vi "PmuError.vi"(8 "error in (no error)":errorcluster, 10 "clPmuImpairRptArray":T1 {"Synx" format="%#_4g"}, 11 "clEvtReportArray":T1 {"Synx" format="%#_4g"}) -> (0 "error out":errorcluster, 3 "Results":dbl[][](array[numeric]))   [LabVIEW 2017, in "OutputToFilePlugins.lvlib" / "OutputToFileBasePlugin.lvclass"]
uses:
  OutputToFileBasePlugin.lvclass
  EventPlugins/EventPluginBaseClass/TypeDefs/clEvtReportArray.ctl
  EventPlugins/EventPluginBaseClass/TypeDefs/clEvtReport.ctl
  <vilib>/ptbypt/NI_PtbyPt.lvlib
  EventPlugins/EventPluginBaseClass/EventPluginBaseClass.lvclass
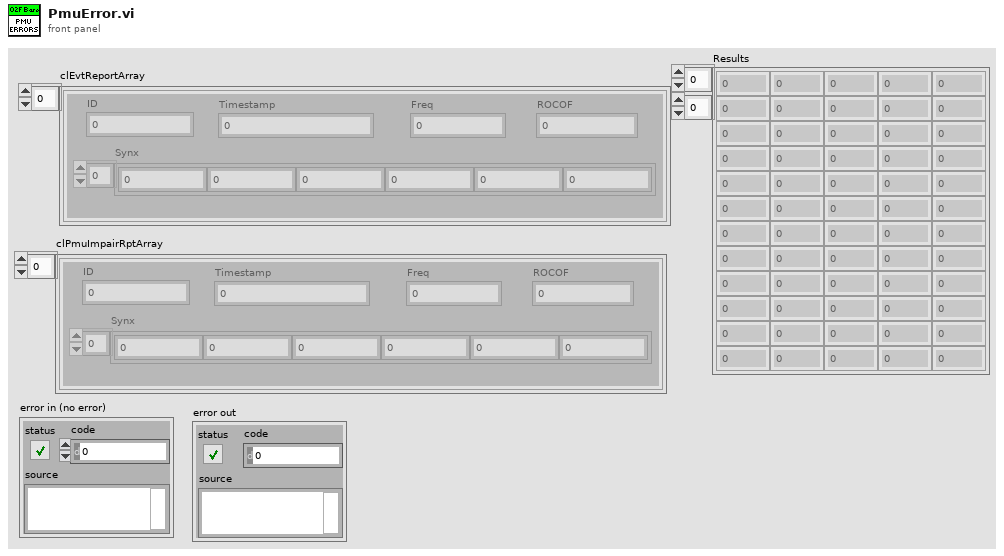
[diagram p1: front panel]
types:
  T1 = typedef "EventPlugins.lvlib/EventPluginBaseClass.lvclass/clEvtReportArray.ctl" = T2[]
  T2 = typedef "EventPlugins.lvlib/EventPluginBaseClass.lvclass/clEvtReport.ctl" = cluster{"Timestamp":dbl, "Synx":cdb[], "Freq":dbl, "ROCOF":dbl, "ID":i16}
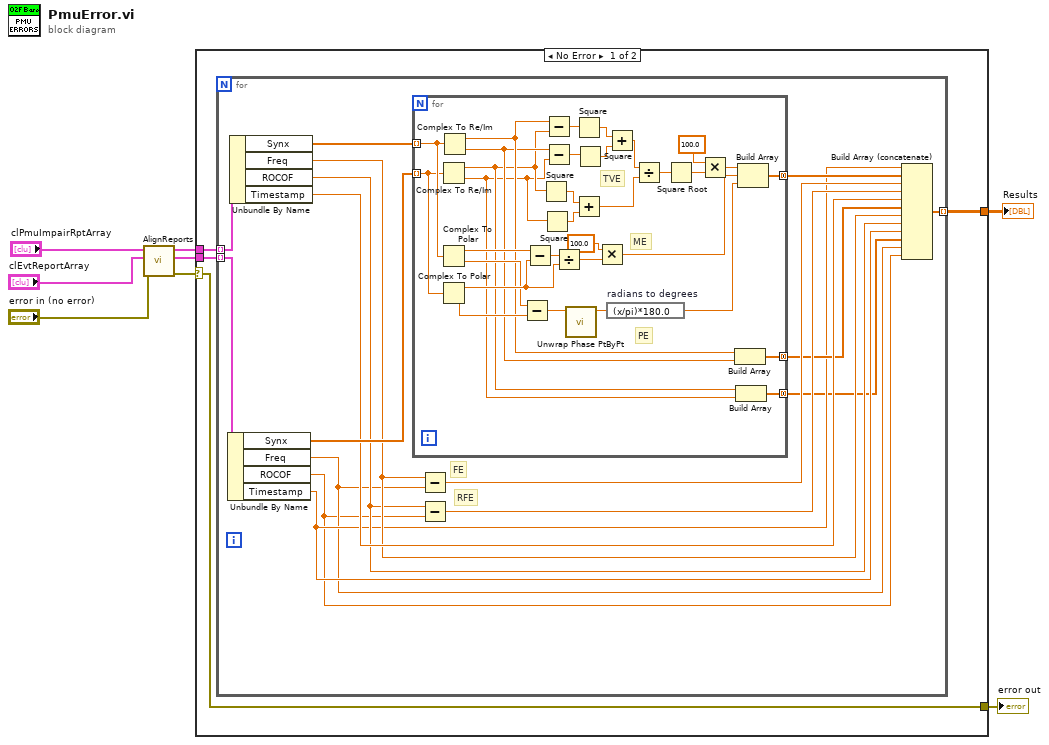
[diagram p0: block diagram]
diagram:
  n1 = call "AlignReports.vi"("error in (no error)"="error in (no error)", "clPmuImpairRptArray"="clEvtReportArray", "clEvtReportArray"="clPmuImpairRptArray") -> ("error out"=w2:errorcluster, "clPmuImpairRptArray"=w6:T1, "clEvtReportArray"=w7:T1)  [unwired: 6 in]
  n2 = case shown="No Error" w2 {
    selector: w2 -> [w9 w61]
    tunnel: w7 -> [w12 _]
    tunnel: w6 -> [w11 _]
    tunnel: [w10 _] -> w3
    tunnel: [w9 w61] -> w1
    frame No Error {
      n3 = for {
        tunnel: w12 -> [w28] mode=indexing
        tunnel: w11 -> [w27] mode=indexing
        tunnel: [w22] -> w10 mode=indexing
        # "RFE"
        # "FE"
        n4 = Unbundle By Name(w27) -> ("Synx"=w26:cdb[], "Freq"=w14:dbl, "ROCOF"=w13:dbl, "Timestamp"=w16:dbl)
        n5 = Unbundle By Name(w28) -> ("Synx"=w20:cdb[], "Freq"=w18:dbl, "ROCOF"=w17:dbl, "Timestamp"=w21:dbl)
        n6 = for {
          tunnel: w20 -> [w52] mode=indexing
          tunnel: w26 -> [w51] mode=indexing
          tunnel: [w36] -> w25 mode=concatenating
          tunnel: [w35] -> w19 mode=concatenating
          tunnel: [w30] -> w15 mode=concatenating
          # "PE"
          # "ME"
          # "TVE"
          n7 = Complex To Re/Im(x + iy=w51) -> (x=w32:dbl, y=w31:dbl)
          n8 = Complex To Polar(r * e^(i*theta)=w52) -> (r=w50:dbl, theta=w43:dbl)
          n9 = Complex To Polar(r * e^(i*theta)=w51) -> (r=w46:dbl, theta=w42:dbl)
          n10 = Complex To Re/Im(x + iy=w52) -> (x=w34:dbl, y=w33:dbl)
          n11 = Subtract(x=w43, y=w42) -> (x-y=w41:dbl)
          n12 = Subtract(x=w50, y=w46) -> (x-y=w47:dbl)
          n13 = Square(x=w32) -> (x^2=w57:dbl)
          n14 = Square(x=w31) -> (x^2=w58:dbl)
          n15 = Subtract(x=w34, y=w32) -> (x-y=w60:dbl)
          n16 = Subtract(x=w33, y=w31) -> (x-y=w59:dbl)
          n17 = Divide(x=w47, y=w46) -> (x/y=w45:dbl)
          n18 = call <vilib>:"Unwrap Phase PtByPt.vi"("phase"=w41) -> ("unwrapped phase"=w40:dbl)  [unwired: 10 in]
          n19 = Square(x=w60) -> (x^2=w55:dbl)
          n20 = Add(x=w57, y=w58) -> (x+y=w53:dbl)
          n21 = Square(x=w59) -> (x^2=w56:dbl)
          n22 = Multiply(x=100.0, y=w45) -> (x*y=w38:dbl)
          n23 = Add(x=w55, y=w56) -> (x+y=w54:dbl)
          n24 = expression code="(x/pi)*180.0" "radians to degrees"(w40) -> (w37:dbl)
          n25 = Divide(x=w54, y=w53) -> (x/y=w49:dbl)
          n26 = Square Root(x=w49) -> (sqrt(x)=w29:dbl)
          n27 = Multiply(x=100.0, y=w29) -> (x*y=w39:dbl)
          n28 = Build Array(w34, w33) -> (w35:dbl[])
          n29 = Build Array(w32, w31) -> (w30:dbl[])
          n30 = Build Array(w39, w38, w37) -> (w36:dbl[])
        }
        n31 = Subtract(x=w18, y=w14) -> (x-y=w24:dbl)
        n32 = Subtract(x=w17, y=w13) -> (x-y=w23:dbl)
        n33 = Build Array (concatenate)(w16, w25, w24, w23, w21, w19, w18, w17, w16, w15, w14, w13) -> (w22:dbl[])
      }
    }
    frame Error {
    }
  }
  "Results" <- w3
  "error out" <- w1
